vi "BT 打印全流程2018.vi"(0 "文件路径":path, 1 "BT 具名数据源名称":string[](array[string]), 2 "输入内容":string[](array[string]), 3 "error in (no error)":errorcluster caption="错误输入（无错误）") -> (10 "error out":errorcluster caption="错误输出")   [LabVIEW 2018]
panel:
  in  "BarTender.IBtApplication":refnum<k7>
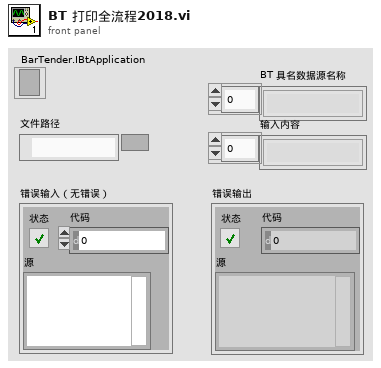
[diagram p1: front panel]
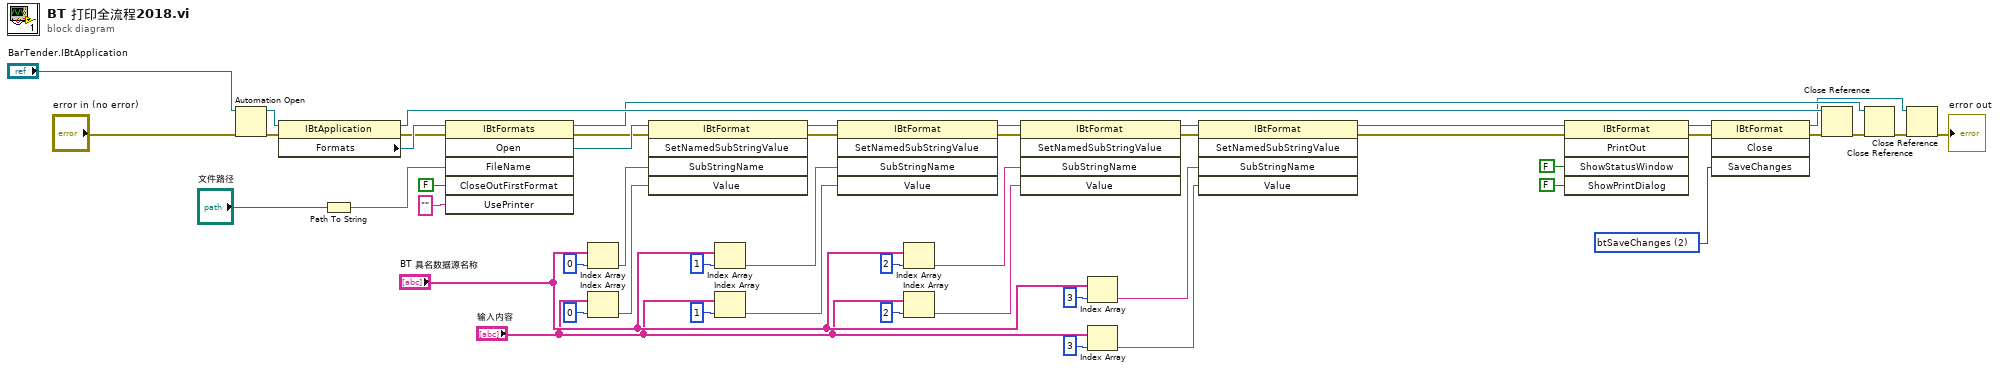
[diagram p0: block diagram]
diagram:
  w37 = 2 items=["btPromptSave", "btDoNotSaveChanges", "btSaveChanges"] ("SaveChanges")
  n1 = Automation Open(error in (no error)="error in (no error)", Automation Refnum="BarTender.IBtApplication") -> (Automation Refnum=w49:refnum<k7>, error out=w48:errorcluster)  [unwired: 2 in]
  n2 = property class="IBtApplication"(reference=w49, error in=w48) -> (reference out=w43:refnum<k7>, error out=w44:errorcluster, "Formats"=w47:refnum<k7>)
  n3 = Path To String(path="文件路径") -> (string=w39:string)
  n4 = invoke class="IBtFormats" method="Open"(reference=w47, error in=w44, "FileName"=w39, "CloseOutFirstFormat"=FALSE, "UsePrinter"="") -> (reference out=w42:refnum<k7>, error out=w27:errorcluster, "Open"=w28:refnum<k7>)  [unwired: 1 in, 3 out]
  n5 = Index Array(array="BT 具名数据源名称", index=0) -> (element=w19:string)
  n6 = Index Array(array="输入内容", index=0) -> (element=w18:string)
  n7 = invoke class="IBtFormat" method="SetNamedSubStringValue"(reference=w28, error in=w27, "SubStringName"=w19, "Value"=w18) -> (reference out=w26:refnum<k7>, error out=w23:errorcluster)  [unwired: 1 in, 3 out]
  n8 = Index Array(array="BT 具名数据源名称", index=1) -> (element=w8:string)
  n9 = Index Array(array="输入内容", index=1) -> (element=w7:string)
  n10 = invoke class="IBtFormat" method="SetNamedSubStringValue"(reference=w26, error in=w23, "SubStringName"=w8, "Value"=w7) -> (reference out=w25:refnum<k7>, error out=w22:errorcluster)  [unwired: 1 in, 3 out]
  n11 = Index Array(array="BT 具名数据源名称", index=2) -> (element=w6:string)
  n12 = Index Array(array="输入内容", index=2) -> (element=w5:string)
  n13 = invoke class="IBtFormat" method="SetNamedSubStringValue"(reference=w25, error in=w22, "SubStringName"=w6, "Value"=w5) -> (reference out=w24:refnum<k7>, error out=w21:errorcluster)  [unwired: 1 in, 3 out]
  n14 = Index Array(array="BT 具名数据源名称", index=3) -> (element=w4:string)
  n15 = Index Array(array="输入内容", index=3) -> (element=w3:string)
  n16 = invoke class="IBtFormat" method="SetNamedSubStringValue"(reference=w24, error in=w21, "SubStringName"=w4, "Value"=w3) -> (reference out=w2:refnum<k7>, error out=w1:errorcluster)  [unwired: 1 in, 3 out]
  n17 = invoke class="IBtFormat" method="PrintOut"(reference=w2, error in=w1, "ShowStatusWindow"=FALSE, "ShowPrintDialog"=FALSE) -> (reference out=w30:refnum<k7>, error out=w29:errorcluster)  [unwired: 1 in, 3 out]
  n18 = invoke class="IBtFormat" method="Close"(reference=w30, error in=w29, "SaveChanges"=w37) -> (reference out=w36:refnum<k7>, error out=w35:errorcluster)  [unwired: 1 in, 2 out]
  n19 = Close Reference(reference=w43, error in (no error)=w35) -> (error out=w41:errorcluster)
  n20 = Close Reference(reference=w42, error in (no error)=w41) -> (error out=w34:errorcluster)
  n21 = Close Reference(reference=w36, error in (no error)=w34) -> (error out=→"error out":errorcluster)
